vi "Логи_БарометрМагнитометр.vi"() -> ()   [LabVIEW 2013]
panel:
  in  "Tab Control":enum32{"Магнитометр", "T и F", "Барометр"}(tab)
  out "?":cluster{dbl[], dbl[]}[](graph)
  out "?":cluster{dbl[], dbl[]}[](graph)
  out "baro":cluster{dbl[], dbl[]}[](graph)
  out "ID параметров":u8[](array[numeric])
  out "Длина заголовка":i32
  out "Заголовок":string
  out "Количество параметров":u8
  out "size (in bytes)":i64
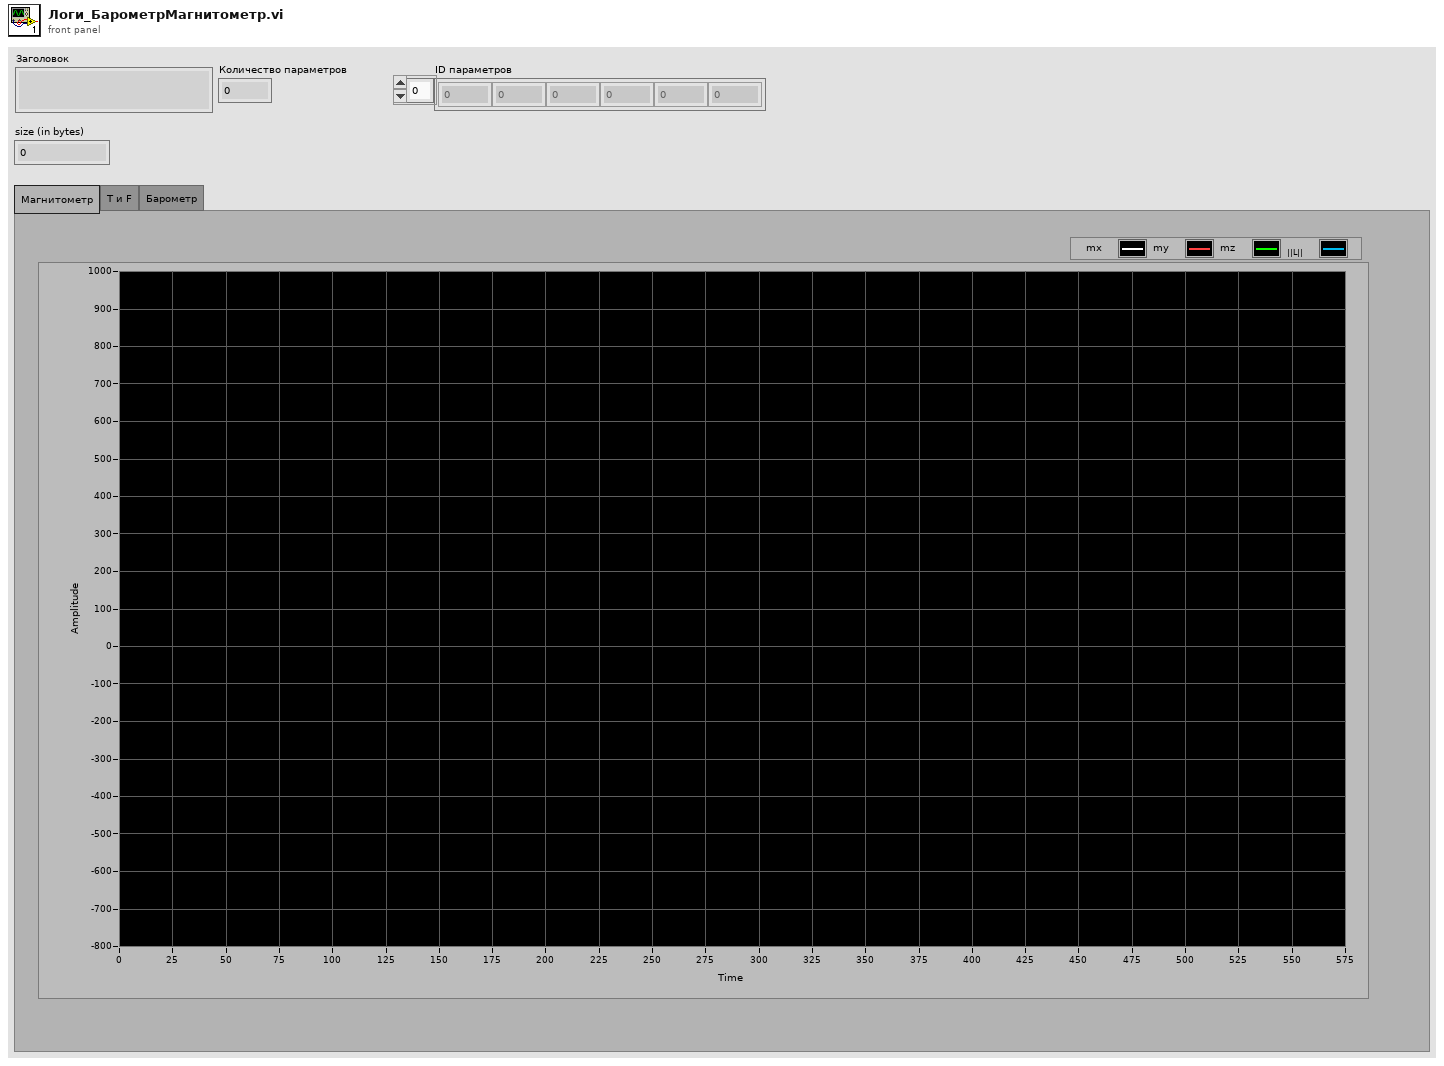
[diagram p1: front panel]
types:
  T1 = enum16{"open", "replace", "create", "open or create", "replace or create", "replace or create with confirmation"}
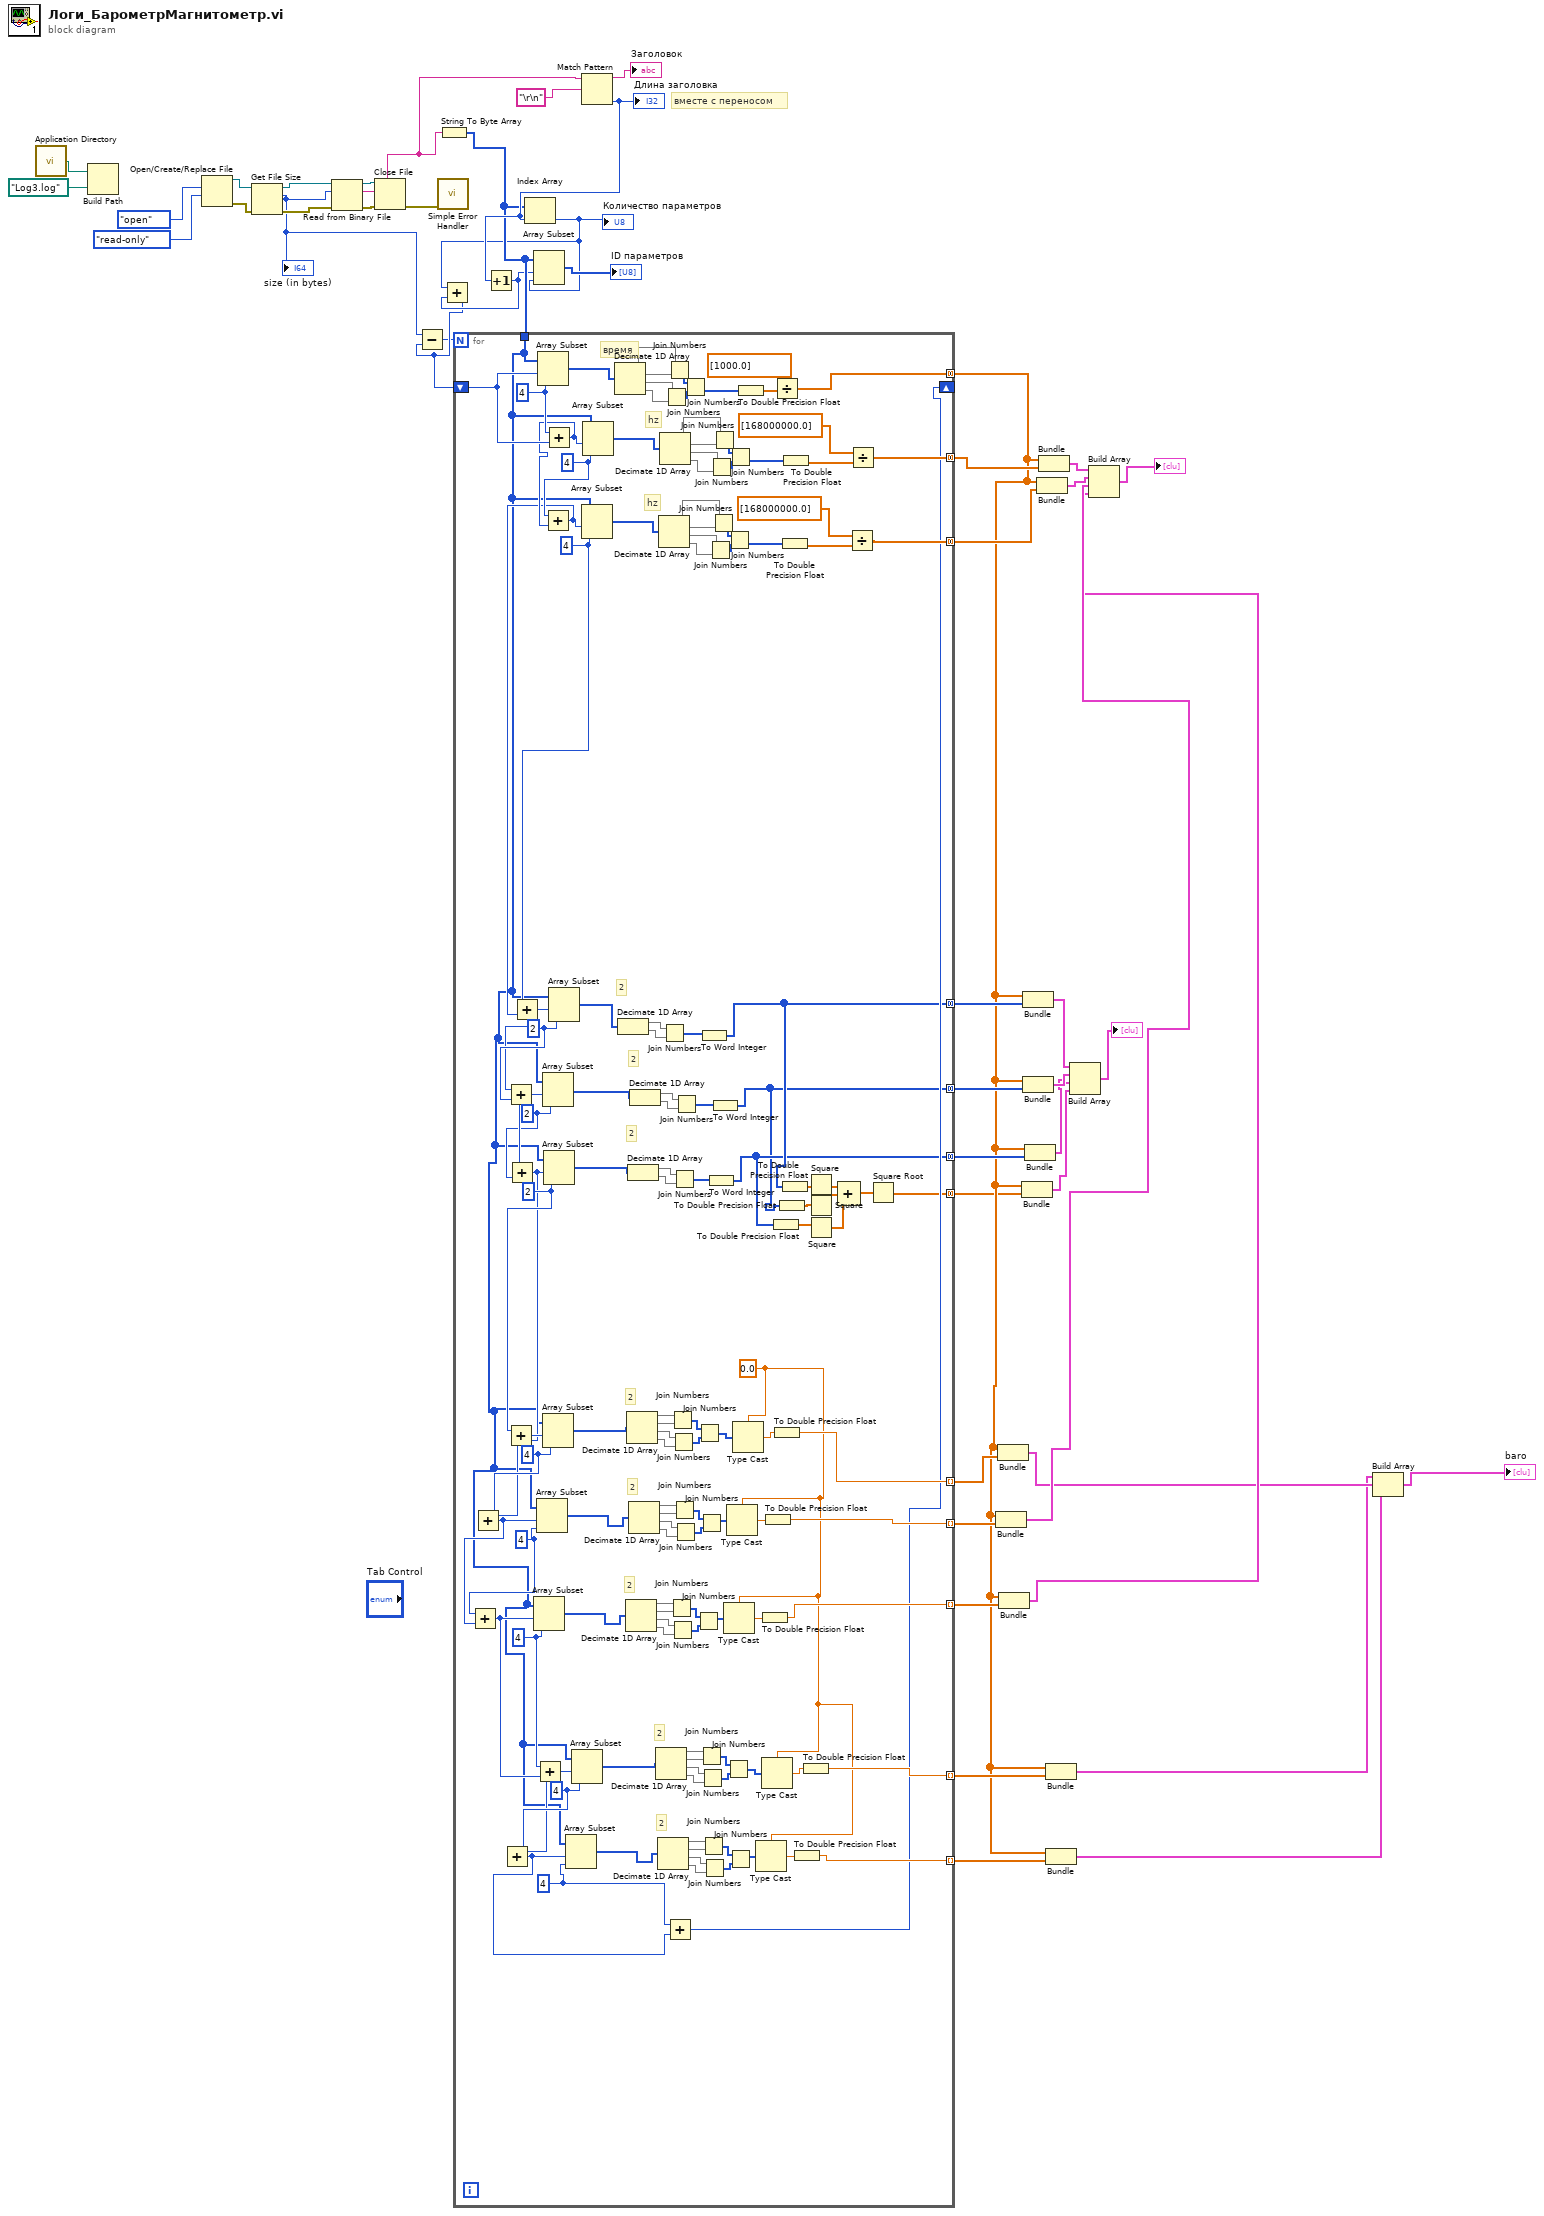
[diagram p0: block diagram]
diagram:
  # "вместе с переносом"
  n1 = call <vilib>:"Application Directory.vi"() -> ("Application Directory"=w45:path)
  n2 = Build Path(base path=w45, name or relative path=path "Log3.log" ("default name")) -> ()  [unwired: 1 out]
  n3 = Open/Create/Replace File(operation (0:open)=T1."open", access (0:read/write)=enum16{"read/write", "read-only", "write-only"}."read-only") -> (refnum out=w42:refnum<file>, error out=w40:errorcluster)  [unwired: 4 in, 1 out]
  n4 = Get File Size(file=w42, error in=w40) -> (refnum out=w41:refnum<file>, size (in bytes)=w32:i64, 0:w39:errorcluster)
  "size (in bytes)" <- w32
  n5 = Read from Binary File(8:w39, 10:w32, 11:w41) -> (0:w43:errorcluster, 2:w38:string, 3:w44:refnum<file>)  [unwired: 3 in, 1 out]
  n6 = Close File(refnum=w44, error in=w43) -> (error out=w48:errorcluster)  [unwired: 1 out]
  n7 = call <vilib>:"Simple Error Handler.vi"("error in (no error)"=w48) -> ()  [unwired: 4 in, 5 out]
  n8 = String To Byte Array(string=w38) -> (unsigned byte array=w33:u8[])
  n9 = Match Pattern(string=w38, regular expression="\r\n" ("format string")) -> (before substring=→"Заголовок":string, offset past match=w35:i32)  [unwired: 1 in, 2 out]
  "Длина заголовка" <- w35
  n10 = Increment(x=w35) -> (x+1=w30:i32)
  n11 = Index Array(array=w33, index=w35) -> (element=w31:u8)
  "Количество параметров" <- w31
  n12 = Add(x=w31, y=w30) -> (x+y=w29:i32)
  n13 = Subtract(x=w32, y=w29) -> (x-y=w28:i64)
  n14 = for {
    N: w28 -> [_]
    tunnel: w33 -> [w64]
    shift-right: [w62] -> _
    shift-left: w29 -> [w113]
    tunnel: [w137] -> w22 mode=indexing
    tunnel: [w136] -> w21 mode=indexing
    tunnel: [w124] -> w17 mode=concatenating
    tunnel: [w110] -> w16 mode=concatenating
    tunnel: [w109] -> w3 mode=concatenating
    tunnel: [w92] -> w14 mode=indexing
    tunnel: [w69] -> w12 mode=indexing
    tunnel: [w68] -> w11 mode=indexing
    tunnel: [w53] -> w10 mode=concatenating
    tunnel: [w50] -> w9 mode=concatenating
    tunnel: [w51] -> w8 mode=concatenating
    tunnel: [w55] -> w2 mode=concatenating
    w61 = 4 ("length")
    w91 = 4 ("length")
    w71 = 4 ("length")
    w105 = 4 ("length")
    w112 = 4 ("length")
    w63 = sgl 0.0
    w93 = 4 ("length")
    w157 = 4 ("length")
    w108 = 2 ("length")
    w177 = 2 ("length")
    w179 = 2 ("length")
    w127 = 4 ("length")
    # "2"
    # "2"
    # "2"
    # "hz"
    # "hz"
    # "2"
    # "2"
    # "2"
    # "2"
    # "2"
    # "время"
    n15 = Array Subset(array=w64, index=w113, length=w127) -> (w169:u8[])
    n16 = Add(x=w127, y=w113) -> (x+y=w111:i32)
    n17 = Add(x=w112, y=w111) -> (x+y=w104:i32)
    n18 = Add(x=w105, y=w104) -> (x+y=w106:i32)
    n19 = Add(x=w106, y=w179) -> (x+y=w178:i32)
    n20 = Add(x=w178, y=w177) -> (x+y=w107:i32)
    n21 = Add(x=w108, y=w107) -> (x+y=w156:i32)
    n22 = Add(x=w156, y=w157) -> (x+y=w94:i32)
    n23 = Add(x=w93, y=w94) -> (x+y=w70:i32)
    n24 = Array Subset(array=w64, index=w70, length=w71) -> (w97:u8[])
    n25 = Add(x=w71, y=w70) -> (x+y=w90:i32)
    n26 = Add(x=w90, y=w91) -> (x+y=w60:i32)
    n27 = Array Subset(array=w64, index=w94, length=w93) -> (w142:u8[])
    n28 = Array Subset(array=w64, index=w178, length=w177) -> (w162:u8[])
    n29 = Array Subset(array=w64, index=w156, length=w157) -> (w149:u8[])
    n30 = Array Subset(array=w64, index=w107, length=w108) -> (w159:u8[])
    n31 = Array Subset(array=w64, index=w106, length=w179) -> (w170:u8[])
    n32 = Array Subset(array=w64, index=w60, length=w61) -> (w76:u8[])
    n33 = Array Subset(array=w64, index=w90, length=w91) -> (w83:u8[])
    n34 = Array Subset(array=w64, index=w104, length=w105) -> (w117:u8[])
    n35 = Array Subset(array=w64, index=w111, length=w112) -> (w129:u8[])
    n36 = Decimate 1D Array(w169) -> (w172:u8[], w173:u8[], w174:u8[], w175:u8[])
    n37 = Decimate 1D Array(w170) -> (w166:u8[], w165:u8[])
    n38 = Decimate 1D Array(w97) -> (w102:u8[], w103:u8[], w101:u8[], w100:u8[])
    n39 = Decimate 1D Array(w149) -> (w154:u8[], w155:u8[], w153:u8[], w152:u8[])
    n40 = Decimate 1D Array(w159) -> (w161:u8[], w160:u8[])
    n41 = Decimate 1D Array(w142) -> (w147:u8[], w148:u8[], w146:u8[], w145:u8[])
    n42 = Decimate 1D Array(w162) -> (w164:u8[], w163:u8[])
    n43 = Decimate 1D Array(w83) -> (w88:u8[], w89:u8[], w87:u8[], w86:u8[])
    n44 = Decimate 1D Array(w76) -> (w81:u8[], w82:u8[], w80:u8[], w79:u8[])
    n45 = Decimate 1D Array(w117) -> (w119:u8[], w120:u8[], w121:u8[], w122:u8[])
    n46 = Decimate 1D Array(w129) -> (w131:u8[], w132:u8[], w133:u8[], w134:u8[])
    n47 = Join Numbers(hi=w166, lo=w165) -> ((hi.lo)=w67:u16[])
    n48 = Join Numbers(hi=w174, lo=w175) -> ((hi.lo)=w171:u16[])
    n49 = Join Numbers(hi=w172, lo=w173) -> ((hi.lo)=w176:u16[])
    n50 = Add(x=w61, y=w60) -> (x+y=w62:i32)
    n51 = Join Numbers(hi=w102, lo=w103) -> ((hi.lo)=w99:u16[])
    n52 = Join Numbers(hi=w154, lo=w155) -> ((hi.lo)=w151:u16[])
    n53 = Join Numbers(hi=w101, lo=w100) -> ((hi.lo)=w98:u16[])
    n54 = Join Numbers(hi=w153, lo=w152) -> ((hi.lo)=w150:u16[])
    n55 = Join Numbers(hi=w161, lo=w160) -> ((hi.lo)=w65:u16[])
    n56 = Join Numbers(hi=w147, lo=w148) -> ((hi.lo)=w144:u16[])
    n57 = Join Numbers(hi=w146, lo=w145) -> ((hi.lo)=w143:u16[])
    n58 = Join Numbers(hi=w164, lo=w163) -> ((hi.lo)=w66:u16[])
    n59 = Join Numbers(hi=w176, lo=w171) -> ((hi.lo)=w158:u32[])
    n60 = Join Numbers(hi=w99, lo=w98) -> ((hi.lo)=w95:u32[])
    n61 = Join Numbers(hi=w151, lo=w150) -> ((hi.lo)=w139:u32[])
    n62 = Join Numbers(hi=w144, lo=w143) -> ((hi.lo)=w140:u32[])
    n63 = Join Numbers(hi=w88, lo=w89) -> ((hi.lo)=w85:u16[])
    n64 = Join Numbers(hi=w87, lo=w86) -> ((hi.lo)=w84:u16[])
    n65 = To Word Integer(number=w67) -> (16bit integer=w53:i16[])
    n66 = Join Numbers(hi=w81, lo=w82) -> ((hi.lo)=w78:u16[])
    n67 = Join Numbers(hi=w80, lo=w79) -> ((hi.lo)=w77:u16[])
    n68 = Join Numbers(hi=w121, lo=w122) -> ((hi.lo)=w118:u16[])
    n69 = To Word Integer(number=w65) -> (16bit integer=w51:i16[])
    n70 = Join Numbers(hi=w133, lo=w134) -> ((hi.lo)=w130:u16[])
    n71 = Join Numbers(hi=w119, lo=w120) -> ((hi.lo)=w123:u16[])
    n72 = Join Numbers(hi=w131, lo=w132) -> ((hi.lo)=w135:u16[])
    n73 = To Word Integer(number=w66) -> (16bit integer=w50:i16[])
    n74 = Type Cast(type=w63, x=w95) -> (*(type *) &x=w96:sgl)
    n75 = Join Numbers(hi=w85, lo=w84) -> ((hi.lo)=w73:u32[])
    n76 = Join Numbers(hi=w123, lo=w118) -> ((hi.lo)=w116:u32[])
    n77 = Join Numbers(hi=w135, lo=w130) -> ((hi.lo)=w128:u32[])
    n78 = Join Numbers(hi=w78, lo=w77) -> ((hi.lo)=w74:u32[])
    n79 = Type Cast(type=w63, x=w140) -> (*(type *) &x=w141:sgl)
    n80 = Type Cast(type=w63, x=w139) -> (*(type *) &x=w138:sgl)
    n81 = To Double Precision Float(number=w158) -> (double precision float=w168:dbl[])
    n82 = Type Cast(type=w63, x=w74) -> (*(type *) &x=w75:sgl)
    n83 = To Double Precision Float(number=w96) -> (double precision float=w92:dbl)
    n84 = Type Cast(type=w63, x=w73) -> (*(type *) &x=w72:sgl)
    n85 = To Double Precision Float(number=w141) -> (double precision float=w136:dbl)
    n86 = To Double Precision Float(number=w51) -> (double precision float=w52:dbl[])
    n87 = Divide(x=w168, y=dbl[] [1000.0]) -> (x/y=w109:dbl[])
    n88 = To Double Precision Float(number=w138) -> (double precision float=w137:dbl)
    n89 = To Double Precision Float(number=w50) -> (double precision float=w49:dbl[])
    n90 = To Double Precision Float(number=w116) -> (double precision float=w115:dbl[])
    n91 = To Double Precision Float(number=w53) -> (double precision float=w54:dbl[])
    n92 = To Double Precision Float(number=w128) -> (double precision float=w126:dbl[])
    n93 = To Double Precision Float(number=w75) -> (double precision float=w68:dbl)
    n94 = To Double Precision Float(number=w72) -> (double precision float=w69:dbl)
    n95 = Square(x=w54) -> (x^2=w59:dbl[])
    n96 = Square(x=w49) -> (x^2=w58:dbl[])
    n97 = Square(x=w52) -> (x^2=w57:dbl[])
    n98 = Compound Arithmetic op=ADD(w59, w58, w57) -> (w56:dbl[])
    n99 = Divide(x=dbl[] [168000000.0] ("y"), y=w115) -> (x/y=w110:dbl[])
    n100 = Divide(x=dbl[] [168000000.0] ("y"), y=w126) -> (x/y=w124:dbl[])
    n101 = Square Root(x=w56) -> (sqrt(x)=w55:dbl[])
  }
  n102 = Array Subset(array=w33, index=w30, length=w31) -> (→"ID параметров":u8[])
  n103 = Bundle(w3, w21) -> (w15:cluster{dbl[], dbl[]})  [unwired: 1 in]
  n104 = Bundle(w3, w22) -> (w6:cluster{dbl[], dbl[]})  [unwired: 1 in]
  n105 = Bundle(w3, w14) -> (w13:cluster{dbl[], dbl[]})  [unwired: 1 in]
  n106 = Bundle(w3, w2) -> (w1:cluster{dbl[], dbl[]})  [unwired: 1 in]
  n107 = Bundle(w3, w10) -> (w27:cluster{dbl[], i16[]})  [unwired: 1 in]
  n108 = Bundle(w3, w9) -> (w26:cluster{dbl[], i16[]})  [unwired: 1 in]
  n109 = Bundle(w3, w8) -> (w25:cluster{dbl[], i16[]})  [unwired: 1 in]
  n110 = Bundle(w3, w16) -> (w19:cluster{dbl[], dbl[]})  [unwired: 1 in]
  n111 = Bundle(w3, w17) -> (w20:cluster{dbl[], dbl[]})  [unwired: 1 in]
  n112 = Bundle(w3, w12) -> (w5:cluster{dbl[], dbl[]})  [unwired: 1 in]
  n113 = Bundle(w3, w11) -> (w4:cluster{dbl[], dbl[]})  [unwired: 1 in]
  n114 = Build Array(w27, w26, w25, w1) -> (→"?":cluster{dbl[], dbl[]}[])
  n115 = Build Array(w20, w19, w15, w13) -> (→"?":cluster{dbl[], dbl[]}[])
  n116 = Build Array(w5, w6, w4) -> (→"baro":cluster{dbl[], dbl[]}[])
